vi "Relay Control - Set Physical Channel.vi"(8 "error in (no error)":errorcluster, 9 "relay action (Close Relay)":T2=enum."Close Relay", 10 "Physical Channels":T1[](array[typedef]), 11 "SLSC Switch in":refnum<class "SLSC Switch.lvclass">) -> (0 "error out":errorcluster, 3 "SLSC Switch out":refnum<class "SLSC Switch.lvclass">)   [LabVIEW 2015, in "SLSC Switch.lvclass"]
uses:
  SLSC Switch.lvclass
  slscsl/RelayAction.ctl
  Controls/Physical Channel.ctl
  SLSC Switch.lvclass/SLSC Switch.ctl
  <vilib>/SLSC/Set Phys Chan Property (Bool).vi
  <vilib>/SLSC/Commit Properties for Phys Chans.vi
  <vilib>/SLSC/SLSC.lvlib
  slscsl/slscsl.lvclass
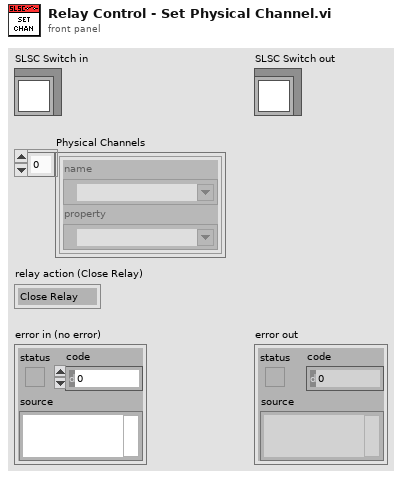
[diagram p1: front panel]
types:
  T1 = typedef "SLSC Switch.lvclass/Physical Channel.ctl" = cluster{"name":refnum<k21>, "property":refnum<k21>}
  T2 = typedef "slscsl.lvclass/RelayAction.ctl" = enum16{"Open Relay", "Close Relay"}
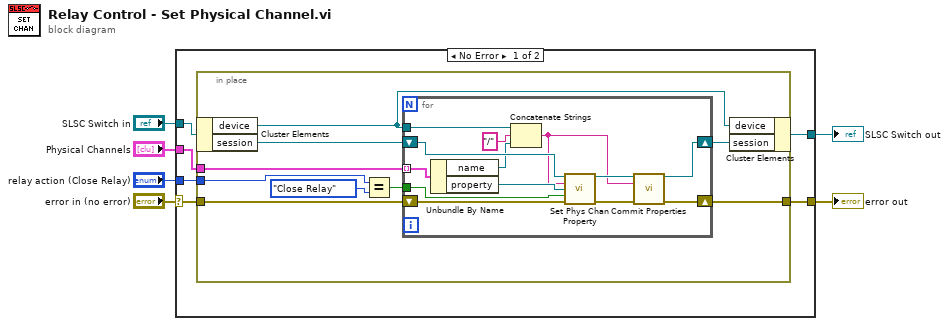
[diagram p0: block diagram]
diagram:
  n1 = case shown="No Error" "error in (no error)" {
    selector: "error in (no error)" -> [w7 w36]
    tunnel: [w11 w36] -> w4
    tunnel: [w10 w35] -> w5
    tunnel: "SLSC Switch in" -> [w9 w35]
    tunnel: "relay action (Close Relay)" -> [w12 _]
    tunnel: "Physical Channels" -> [w8 _]
    frame No Error {
      n2 = in-place {
        in-place-border: w12 -> [w15]
        in-place-border: [w20] -> w11
        in-place-border: w7 -> [w19]
        in-place-border: w8 -> [w17]
        n3 = in-place-cluster #1(w9) -> ("device"=w16:refnum<k21>, "session"=w18:refnum<k21>)
        n4 = Equal?(x=w15, y=RelayAction."Close Relay") -> (x = y?=w13:bool)
        n5 = for {
          tunnel: w13 -> [w34]
          tunnel: w17 -> [w27] mode=indexing
          shift-right: [w30] -> w20
          shift-left: w19 -> [w29]
          shift-right: [w31] -> w21
          shift-left: w18 -> [w28]
          tunnel: w16 -> [w25]
          n6 = Unbundle By Name(w27) -> ("name"=w24:refnum<k21>, "property"=w26:refnum<k21>)
          n7 = Concatenate Strings(w25, "/" ("string"), w24) -> (w23:string)
          n8 = call-poly <vilib>:"Set Phys Chan Property.vi"("session in"=w28, "physical channels"=w23, "property"=w26, "property value"=w34, "error in (no error)"=w29) -> ("session out"=w33:refnum<k21>, "error out"=w32:errorcluster)  [unwired: 9 in]
          n9 = call-poly <vilib>:"Commit Properties.vi"("session in"=w33, "physical channels"=w23, "error in (no error)"=w32) -> ("session out"=w31:refnum<k21>, "error out"=w30:errorcluster)  [unwired: 11 in]
        }
        n10 = in-place-cluster #1("device"=w16, "session"=w21) -> (w10:refnum<class "SLSC Switch.lvclass">)
      }
    }
    frame Error {
    }
  }
  "error out" <- w4
  "SLSC Switch out" <- w5
